vi "CSM.vi"(7 "Name(\"\" to use uuid)":string="csm") -> ()   [LabVIEW 2020]
uses:
  d2b1b62f-1b90-408b-bb7a-e556077d75a7.vi
  8b8ec819-a2be-48ca-834e-c0b9cb0b2cd9.vi
  <userlib>/_NEVSTOP/Communicable State Machine(CSM)/_Support/Common/Format Timestamp.vi
  <userlib>/_NEVSTOP/Communicable State Machine(CSM)/AdvanceAPI/CSM - Revert Arguments-Safe String.vi
  <userlib>/_NEVSTOP/Communicable State Machine(CSM)/_Support/Common/Trim Single line Text.vi
  <userlib>/_NEVSTOP/Communicable State Machine(CSM)/AdvanceAPI/CSM - Make String Arguments Safe.vi
  <userlib>/_NEVSTOP/Communicable State Machine(CSM)/AdvanceAPI/CSM - Break Down Multiple States String.vi
  <userlib>/_NEVSTOP/Communicable State Machine(CSM)/AdvanceAPI/CSM - Compact Multiple States.vi
  <userlib>/_NEVSTOP/Communicable State Machine(CSM)/AdvanceAPI/CSM - Keywords.vi
  <userlib>/_NEVSTOP/Communicable State Machine(CSM)/addons/API-String-Arugments-Support/_Support/Data To API String Arguments.vi
  Global.vi
  <userlib>/_NEVSTOP/Communicable State Machine(CSM)/Communicable State Machine.lvlib
panel:
  out "State History":string
  in  "Init State(\"Macro: Initialize\")":string="Macro: Initialize"
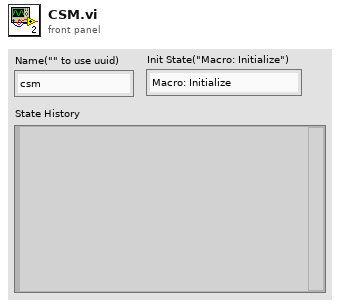
[diagram p1: front panel]
types:
  T1 = enum32{"Invalid", "Standard", "Closed", "Hidden", "Minimized", "Maximized"}
  T2 = enum32{"invalid app kind", "Development System", "Run Time System", "Student Edition", "Embedded LabVIEW", "Evaluation", "Custom"}
  T3 = typedef "Communicable State Machine.lvlib/_CSM_Response Source Message.ctl" = cluster{"‘State":string, "’Arguments":string, "’Error":errorcluster}
  T4 = cluster{"Current VI Reference":refnum<vi>, "Close Panel on Exit?":bool}
  T5 = cluster{"Core":cluster{"Current VI Reference":refnum<vi>, "Close Panel on Exit?":bool}, "num":i32}
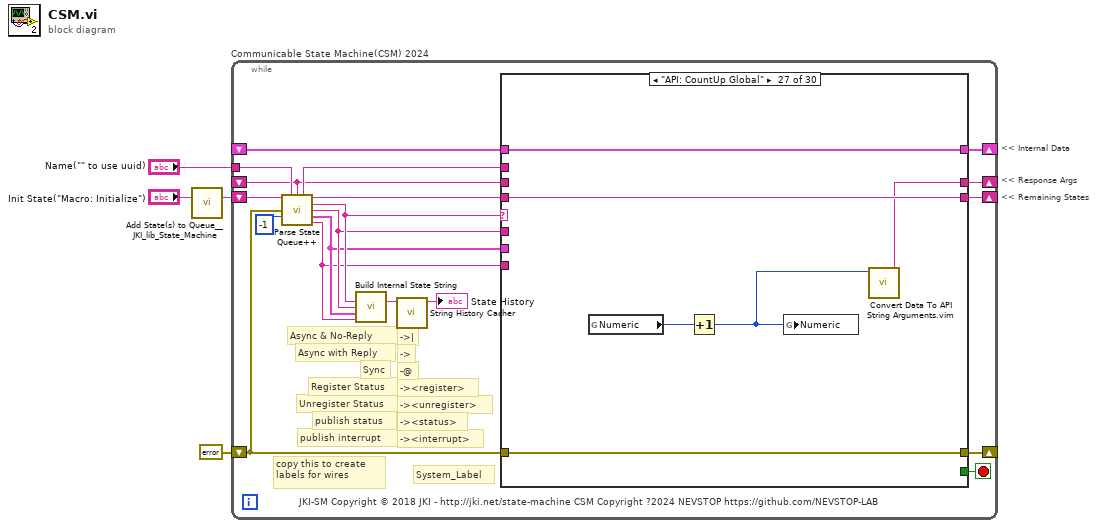
[diagram p0: block diagram]
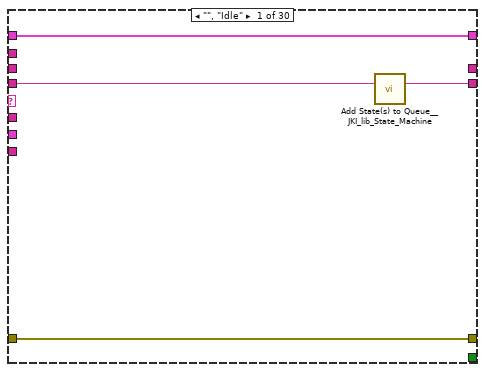
[diagram p2: hidden frame]
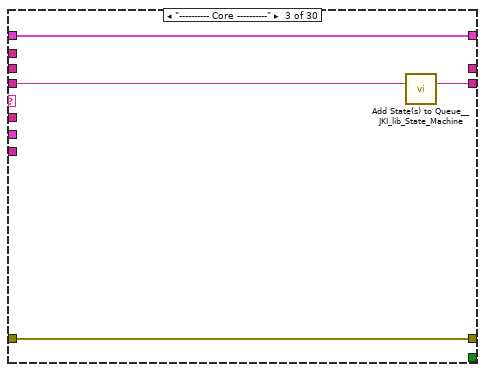
[diagram p4: hidden frame]
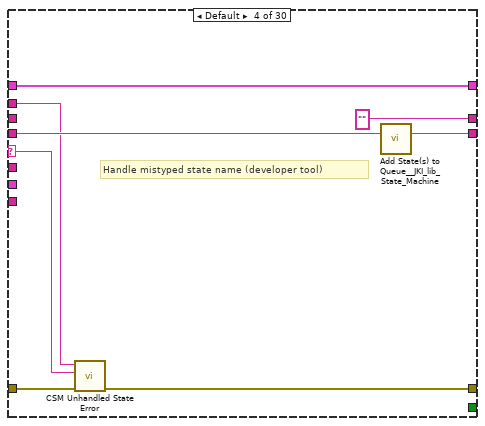
[diagram p5: hidden frame]
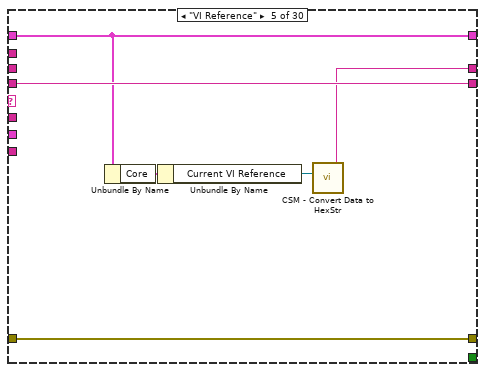
[diagram p6: hidden frame]
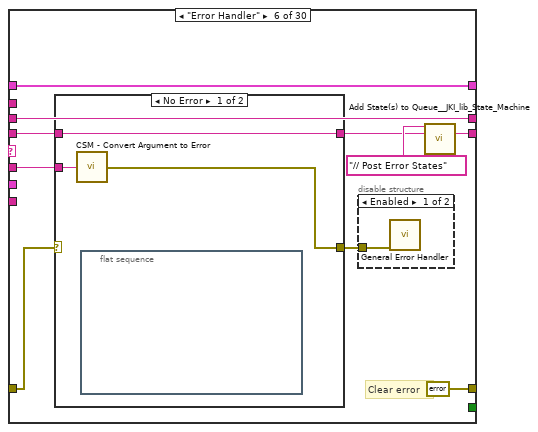
[diagram p7: hidden frame]
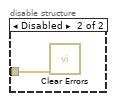
[diagram p8: hidden frame]
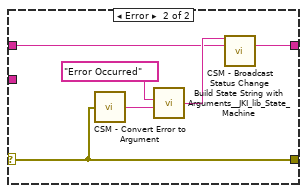
[diagram p9: hidden frame]
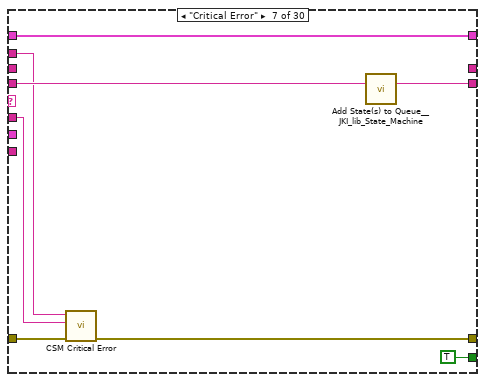
[diagram p10: hidden frame]
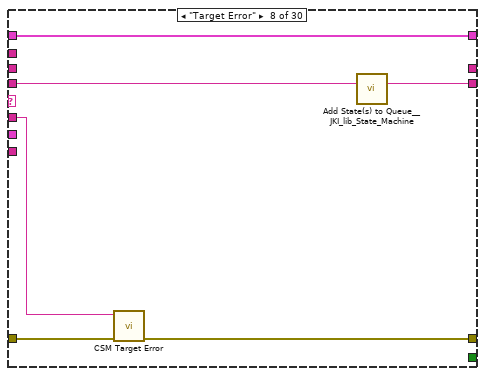
[diagram p11: hidden frame]
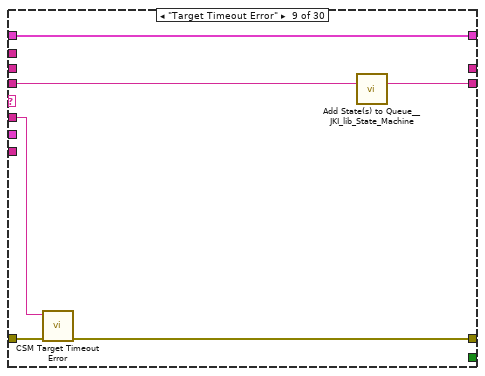
[diagram p12: hidden frame]
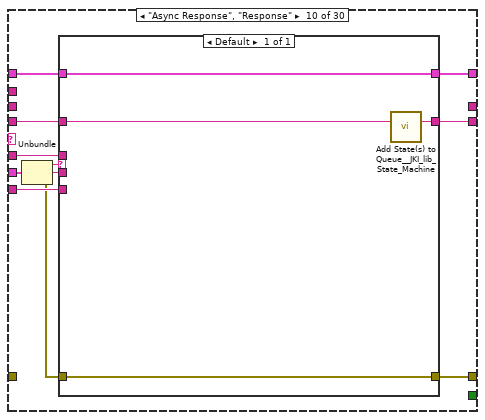
[diagram p13: hidden frame]
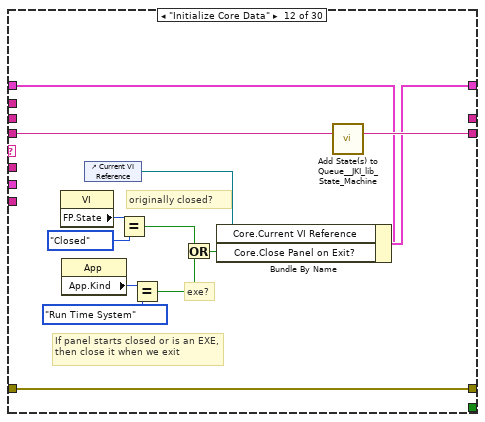
[diagram p15: hidden frame]
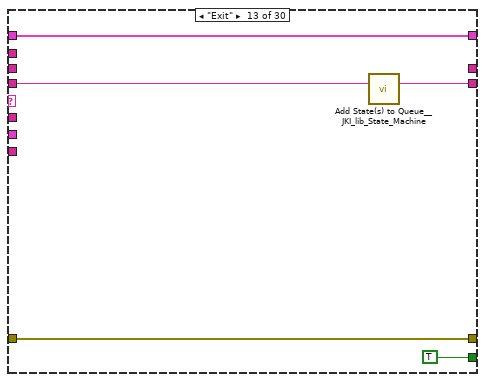
[diagram p16: hidden frame]
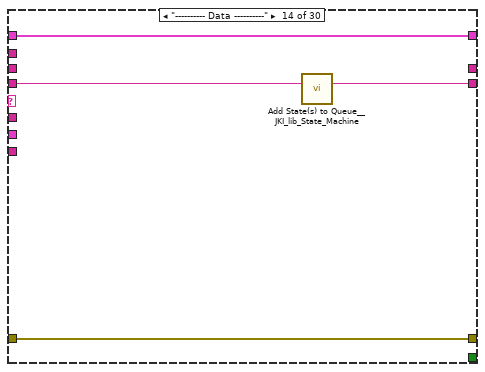
[diagram p17: hidden frame]
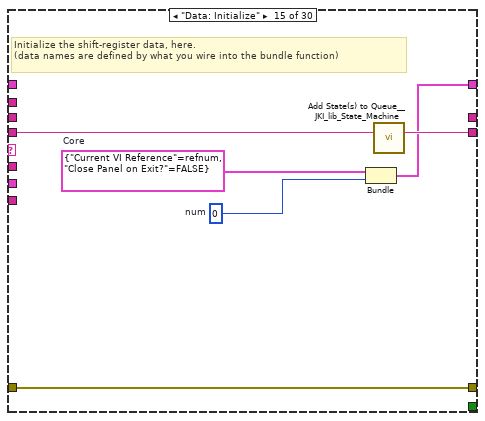
[diagram p18: hidden frame]
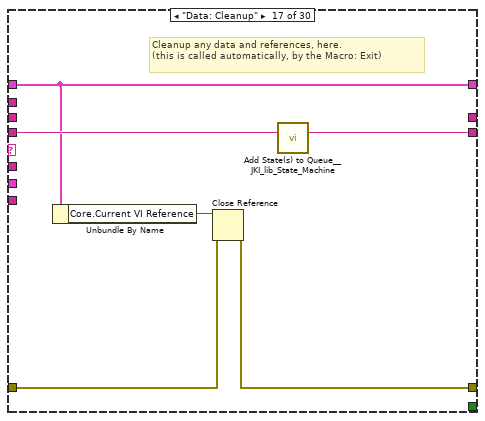
[diagram p20: hidden frame]
diagram:
  # "<< Internal Data"
  # "<< Response Args"
  # "<< Remaining States"
  n1 = call <vilib>:"Add State(s) to Queue__JKI_lib_State_Machine.vi"("State(s) in (\"\")"="Init State(\"Macro: Initialize\")") -> ("States Out"=w1:string)  [unwired: 14 in]
  n2 = while "Communicable State Machine(CSM) 2024" {
    shift-right: [w18] -> _
    shift-left: _ -> [w17]
    shift-right: [w21] -> _
    shift-left: errorcluster {"status"=FALSE, "code"=0, "source"=""} ("error out") -> [w16]
    shift-right: [w20] -> _
    shift-left: w1 -> [w22]
    tunnel: "Name(\"\" to use uuid)" -> [w14]
    shift-right: [w15] -> _
    shift-left: _ -> [w6]
    stop <- w19 stop-if-true
    # "-><interrupt>"
    # "-><status>"
    # "-><unregister>"
    # "-><register>"
    # "-@"
    # "->"
    # "->|"
    # "publish interrupt"
    # "publish status"
    # "Unregister Status"
    # "Register Status"
    # "Sync"
    # "Async with Reply"
    # "Async & No-Reply"
    # "copy this to create labels for wires"
    # "System_Label"
    # "JKI-SM Copyright © 2018 JKI - http://jki.net/state-machine CSM Copyright ?2024 NEVSTOP https://github.com/NEVSTOP-LAB"
    n3 = call <userlib>:"Parse State Queue++.vi"("State Queue"=w22, "Name(\"\" to use uuid)"=w14, "Response Arguments"=w6, "Previous Error"=w16, "Dequeue Timeout(0ms)"=-1 ("Timeout")) -> ("Name Used"=w7:string, "Remaining States"=w23:string, "Current State"=w11:string, "Arguments"=w10:string, ">> Response Source Message >>"=w9:T3, ">> Source CSM >>"=w8:string)  [unwired: 5 in]
    n4 = call <userlib>:"Build Internal State String.vi"("State"=w11, "Arguments (\"\")"=w10, ">> Response Source Message >>"=w9, "Source (\"\")"=w8) -> ("State with Arguments"=w12:string)  [unwired: 11 in]
    n5 = call <userlib>:"String History Cacher.vi"("String"=w12) -> ("String Cache"=→"State History":string)  [unwired: 10 in]
    n6 = case shown="\"API: CountUp Global\"" w11 {
      selector: w11 -> [_ _ _ w37 _ _ _ _ _ _ _ _ _ _ _ _ _ _ _ _ _ _ _ _ _ _ _ _ _ _]
      tunnel: w23 -> [w24 w29 w34 w41 w47 w54 w75 w81 w87 w95 w106 w120 w125 w129 w135 w137 w144 w148 w152 w158 w173 w242 w247 w254 w256 w263 w269 w274 w278 w282]
      tunnel: w10 -> [_ _ _ _ _ w53 w71 w80 w85 w94 _ _ _ _ _ _ _ _ _ w153 w167 _ _ _ _ _ _ _ _ _]
      tunnel: w17 -> [w25 w28 w31 w39 w46 w57 w76 w82 w88 w97 w105 w113 w123 w126 _ w136 w139 w145 w150 w156 w169 w239 w244 w251 w255 w262 w268 w271 w275 w279]
      tunnel: [w26 w30 w32 w35 w48 errorcluster {"status"=FALSE, "code"=0, "source"=""} ("error out") w72 w78 w84 w100 w107 w117 w122 w127 w132 w138 w140 w146 w149 w154 w170 w240 w245 w252 w257 w264 w270 w272 w276 w280] -> w21
      tunnel: w16 -> [w26 w30 w32 w42 w48 w55 w77 w79 w86 _ w107 w117 w122 w127 w132 w138 w141 w146 w149 w155 w171 w240 w245 w252 w257 w264 w270 w272 w276 w280]
      tunnel: [w27 w29 w33 w40 w47 w50 w74 w83 w89 w96 w106 w119 w124 w128 w134 w137 w143 w147 w151 w157 w172 w241 w246 w253 w256 w263 w269 w273 w277 w281] -> w20
      tunnel: [_ _ _ _ _ _ TRUE _ _ _ _ _ TRUE _ _ _ _ _ _ _ _ _ _ _ _ _ _ _ _ _] -> w19
      tunnel: [w25 w28 w31 w39 w46 w57 w76 w82 w88 w98 w105 w118 w123 w126 w133 w136 w139 w145 w150 w156 w169 w239 w244 w251 w255 w260 w268 w271 w275 w279] -> w18
      tunnel: w8 -> [_ _ _ _ _ _ _ _ _ w92 _ _ _ _ _ _ _ _ _ _ _ _ _ _ _ _ _ _ _ _]
      tunnel: w9 -> [_ _ _ _ _ _ _ _ _ w99 _ _ _ _ _ _ _ _ _ _ _ _ _ _ _ _ _ _ _ _]
      tunnel: [_ _ _ "" w43 w49 _ _ _ _ _ _ _ _ _ _ _ _ _ _ _ _ _ _ _ w258 w267 _ _ _] -> w15
      tunnel: w7 -> [_ _ _ w36 _ _ w70 _ _ _ _ _ _ _ _ _ _ _ _ _ _ _ _ _ _ _ _ _ _ _]
      tunnel: w6 -> [_ _ _ _ _ w49 _ _ _ _ _ _ _ _ _ _ _ _ _ _ _ _ _ _ _ _ _ _ _ _]
      frame "", "Idle" {
        n7 = call <vilib>:"Add State(s) to Queue__JKI_lib_State_Machine.vi"("State(s) in (\"\")"=w24) -> ("States Out"=w27:string)  [unwired: 14 in]
      }
      frame "CSM Documentation" {
      }
      frame "---------- Core ----------" {
        n8 = call <vilib>:"Add State(s) to Queue__JKI_lib_State_Machine.vi"("State(s) in (\"\")"=w34) -> ("States Out"=w33:string)  [unwired: 14 in]
      }
      frame Default {
        # "Handle mistyped state name (developer tool)"
        n9 = call <userlib>:"CSM Unhandled State Error.vi"("error in (no error)"=w42, "Current State"=w37, "CSM Name"=w36) -> ("error out"=w35:errorcluster)  [unwired: 8 in]
        n10 = call <vilib>:"Add State(s) to Queue__JKI_lib_State_Machine.vi"("State(s) in (\"\")"=w41) -> ("States Out"=w40:string)  [unwired: 14 in]
      }
      frame "VI Reference" {
        n11 = Unbundle By Name(w46) -> ("Core"=w45:T4)
        n12 = Unbundle By Name(w45) -> ("Current VI Reference"=w44:refnum<vi>)
        n13 = call <userlib>:"CSM - Convert Data to HexStr.vi"("Variant"=w44) -> ("HEX String (0-9,A-F)"=w43:string)  [unwired: 8 in]
      }
      frame "Error Handler" {
        # "Clear error"
        n14 = case shown="No Error" w55 {
          selector: w55 -> [_ w64]
          tunnel: [w63 w66] -> w51
          tunnel: w54 -> [w63 w65]
          tunnel: w53 -> [w62 _]
          tunnel: [w61 w64] -> w56
          frame No Error {
            n15 = call <userlib>:"CSM - Convert Argument to Error.vi"("Argument"=w62) -> ("error"=w61:errorcluster)  [unwired: 4 in]
            n16 = flat-sequence {
              frame #0 {
              }
            }
          }
          frame Error {
            n17 = call <userlib>:"CSM - Convert Error to Argument.vi"("error"=w64) -> ("Argument"=w68:string)  [unwired: 4 in]
            n18 = call <vilib>:"Build State String with Arguments__JKI_lib_State_Machine.vi"("Arguments (\"\")"=w68, "State"="Error Occurred" ("Status with Arguments")) -> ("State with Arguments"=w67:string)  [unwired: 4 in]
            n19 = call <userlib>:"CSM - Broadcast Status Change.vi"("Status with Arguments"=w67, "State Queue"=w65) -> ("Remaining States"=w66:string)  [unwired: 13 in]
          }
        }
        n20 = disable-structure shown="Enabled" {
          disable-tunnel: w56 -> [w59 w60]
          frame Enabled {
            n21 = call <vilib>:"General Error Handler.vi"("error in (no error)"=w59) -> ()  [unwired: 10 in, 5 out]
          }
          frame Disabled {
            n22 = call <vilib>:"Clear Errors.vi"("error in (no error)"=w60) -> ()  [unwired: 5 in, 2 out]
          }
        }
        n23 = call <vilib>:"Add State(s) to Queue__JKI_lib_State_Machine.vi"("State(s) in Front (\"\")"="// Post Error States", "State(s) in (\"\")"=w51) -> ("States Out"=w50:string)  [unwired: 13 in]
      }
      frame "Critical Error" {
        n24 = call <userlib>:"CSM Critical Error.vi"("error in (no error)"=w77, "Arugments(as Reason)"=w71, "CSM Name"=w70) -> ("error out"=w72:errorcluster)  [unwired: 8 in]
        n25 = call <vilib>:"Add State(s) to Queue__JKI_lib_State_Machine.vi"("State(s) in (\"\")"=w75) -> ("States Out"=w74:string)  [unwired: 14 in]
      }
      frame "Target Error" {
        n26 = call <userlib>:"CSM Target Error.vi"("error in (no error)"=w79, "Arguments(as CSM Name)"=w80) -> ("error out"=w78:errorcluster)  [unwired: 9 in]
        n27 = call <vilib>:"Add State(s) to Queue__JKI_lib_State_Machine.vi"("State(s) in (\"\")"=w81) -> ("States Out"=w83:string)  [unwired: 14 in]
      }
      frame "Target Timeout Error" {
        n28 = call <userlib>:"CSM Target Timeout Error.vi"("error in (no error)"=w86, "Arguments(as CSM Name)"=w85) -> ("error out"=w84:errorcluster)  [unwired: 9 in]
        n29 = call <vilib>:"Add State(s) to Queue__JKI_lib_State_Machine.vi"("State(s) in (\"\")"=w87) -> ("States Out"=w89:string)  [unwired: 14 in]
      }
      frame "Async Response", "Response" {
        n30 = Unbundle(w99) -> ("‘State"=w93:string, "’Arguments"=w91:string, "’Error"=w90:errorcluster)
        n31 = case shown="Default" w93 {
          tunnel: [w104] -> w100
          tunnel: w90 -> [w104]
          tunnel: [w103] -> w98
          tunnel: w97 -> [w103]
          tunnel: [w101] -> w96
          tunnel: w95 -> [w102]
          tunnel: w94 -> [_]
          tunnel: w92 -> [_]
          tunnel: w91 -> [_]
          frame Default {
            n32 = call <vilib>:"Add State(s) to Queue__JKI_lib_State_Machine.vi"("State(s) in (\"\")"=w102) -> ("States Out"=w101:string)  [unwired: 14 in]
          }
        }
      }
      frame "Async Message Posted" {
      }
      frame "Initialize Core Data" {
        # "originally closed?"
        # "exe?"
        # "If panel starts closed or is an EXE, then close it when we exit"
        n33 = property class="VI"() -> ("FP.State"=w110:T1)  [unwired: 2 in, 2 out]
        n34 = property class="App"() -> ("App.Kind"=w116:T2)  [unwired: 2 in, 2 out]
        n35 = control-ref of="Current VI Reference"() -> (w111:refnum<vi>)
        n36 = Equal?(x=w110, y=T1."Closed" ("Front Panel Window:State")) -> (x = y?=w108:bool)
        n37 = Equal?(x=w116, y=T2."Run Time System" ("Application:Kind")) -> (x = y?=w114:bool)
        n38 = Or(x=w108, y=w114) -> (x .or. y?=w112:bool)
        n39 = Bundle By Name(cluster=w113, "Core.Current VI Reference"=w111, "Core.Close Panel on Exit?"=w112) -> (w118:T5)
        n40 = call <vilib>:"Add State(s) to Queue__JKI_lib_State_Machine.vi"("State(s) in (\"\")"=w120) -> ("States Out"=w119:string)  [unwired: 14 in]
      }
      frame "Exit" {
        n41 = call <vilib>:"Add State(s) to Queue__JKI_lib_State_Machine.vi"("State(s) in (\"\")"=w125) -> ("States Out"=w124:string)  [unwired: 14 in]
      }
      frame "---------- Data ----------" {
        n42 = call <vilib>:"Add State(s) to Queue__JKI_lib_State_Machine.vi"("State(s) in (\"\")"=w129) -> ("States Out"=w128:string)  [unwired: 14 in]
      }
      frame "Data: Initialize" {
        w130 = T4 {"Current VI Reference"=refnum, "Close Panel on Exit?"=FALSE}  # Core
        w131 = 0  # num
        # "Initialize the shift-register data, here.\n(data names are defined by what you wire into the bundle function)"
        n43 = Bundle("Core"=w130, "num"=w131) -> (w133:T5)  [unwired: 1 in]
        n44 = call <vilib>:"Add State(s) to Queue__JKI_lib_State_Machine.vi"("State(s) in (\"\")"=w135) -> ("States Out"=w134:string)  [unwired: 14 in]
      }
      frame "Data: Update Indicators" {
      }
      frame "Data: Cleanup" {
        # "Cleanup any data and references, here.\n(this is called automatically, by the Macro: Exit)"
        n45 = Unbundle By Name(w139) -> ("Core.Current VI Reference"=w142:refnum<vi>)
        n46 = Close Reference(reference=w142, error in (no error)=w141) -> (error out=w140:errorcluster)
        n47 = call <vilib>:"Add State(s) to Queue__JKI_lib_State_Machine.vi"("State(s) in (\"\")"=w144) -> ("States Out"=w143:string)  [unwired: 14 in]
      }
      frame "---------- UI ----------" {
        n48 = call <vilib>:"Add State(s) to Queue__JKI_lib_State_Machine.vi"("State(s) in (\"\")"=w148) -> ("States Out"=w147:string)  [unwired: 14 in]
      }
      frame "UI: Initialize" {
        n49 = call <vilib>:"Add State(s) to Queue__JKI_lib_State_Machine.vi"("State(s) in (\"\")"=w152) -> ("States Out"=w151:string)  [unwired: 14 in]
      }
      frame "UI: Cursor Set" {
        # "Argument"
        n50 = disable-structure shown="TARGET_TYPE!=Windows" {
          disable-tunnel: w155 -> [w161 w166]
          disable-tunnel: [w160 w166] -> w154
          disable-tunnel: w153 -> [w159 _]
          frame condition #0 (active) {
            n51 = case shown="\"Idle\", Default" w159 {
              tunnel: w161 -> [w163 w165]
              tunnel: [w162 w164] -> w160
              frame "Idle", Default {
                n52 = call <vilib>:"Unset Busy.vi"("error in (no error)"=w163) -> ("error out"=w162:errorcluster)  [unwired: 10 in]
              }
              frame "Busy" {
                n53 = call <vilib>:"Set Busy.vi"("error in (no error)"=w165) -> ("error out"=w164:errorcluster)  [unwired: 9 in, 1 out]
              }
            }
          }
          frame condition #1 {
          }
        }
        n54 = call <vilib>:"Add State(s) to Queue__JKI_lib_State_Machine.vi"("State(s) in (\"\")"=w158) -> ("States Out"=w157:string)  [unwired: 14 in]
      }
      frame "UI: Front Panel State" {
        # "Argument"
        n55 = Unbundle By Name(w169) -> ("Core.Current VI Reference"=w168:refnum<vi>)
        n56 = call <vilib>:"Add State(s) to Queue__JKI_lib_State_Machine.vi"("State(s) in (\"\")"=w173) -> ("States Out"=w172:string)  [unwired: 14 in]
        n57 = case shown="\"Close\", \"Closed\"" w167 {
          tunnel: w171 -> [w179 w194 w205 w218 w231]
          tunnel: [w181 w195 w207 w220 w233] -> w170
          tunnel: w168 -> [w180 w192 w206 w219 w232]
          frame "Open", "Standard", Default {
            w174 = T1."Standard" ("State")
            n58 = property class="VI"(reference=w180, error in=w179) -> (reference out=w177:refnum<vi>, error out=w178:errorcluster, "FP.State"=w176:T1)
            n59 = Not Equal?(x=w176, y=w174) -> (x != y?=w175:bool)
            n60 = case shown="True" w175 {
              tunnel: [w185 w187] -> w181
              tunnel: w178 -> [w184 w187]
              tunnel: w177 -> [w183 _]
              tunnel: w174 -> [w182 _]
              frame True {
                n61 = invoke class="VI" method="FP.Open"(reference=w183, error in=w184, "Activate"=TRUE, "State"=w182) -> (error out=w185:errorcluster)  [unwired: 1 in, 4 out]
              }
              frame False {
              }
            }
          }
          frame "Close", "Closed" {
            n62 = property class="VI"(reference=w192, error in=w194) -> (reference out=w191:refnum<vi>, error out=w193:errorcluster, "FP.State"=w189:T1)
            n63 = Not Equal?(x=w189, y=T1."Closed" ("Front Panel Window:State")) -> (x != y?=w188:bool)
            n64 = case shown="False" w188 {
              tunnel: [w196 w199] -> w195
              tunnel: w193 -> [w196 w198]
              tunnel: w191 -> [_ w197]
              frame False {
              }
              frame True {
                n65 = invoke class="VI" method="FP.Close"(reference=w197, error in=w198) -> (error out=w199:errorcluster)  [unwired: 1 in, 2 out]
              }
            }
          }
          frame "Hidden", "Hide" {
            w200 = T1."Hidden" ("State")
            n66 = property class="VI"(reference=w206, error in=w205) -> (reference out=w203:refnum<vi>, error out=w204:errorcluster, "FP.State"=w202:T1)
            n67 = Not Equal?(x=w202, y=w200) -> (x != y?=w201:bool)
            n68 = case shown="True" w201 {
              tunnel: [w211 w212] -> w207
              tunnel: w204 -> [w210 w212]
              tunnel: w203 -> [w209 _]
              tunnel: w200 -> [w208 _]
              frame True {
                n69 = invoke class="VI" method="FP.Open"(reference=w209, error in=w210, "State"=w208) -> (error out=w211:errorcluster)  [unwired: 2 in, 4 out]
              }
              frame False {
              }
            }
          }
          frame "Minimize", "Minimized" {
            w213 = T1."Minimized" ("State")
            n70 = property class="VI"(reference=w219, error in=w218) -> (reference out=w216:refnum<vi>, error out=w217:errorcluster, "FP.State"=w215:T1)
            n71 = Not Equal?(x=w215, y=w213) -> (x != y?=w214:bool)
            n72 = case shown="True" w214 {
              tunnel: [w224 w225] -> w220
              tunnel: w217 -> [w223 w225]
              tunnel: w216 -> [w222 _]
              tunnel: w213 -> [w221 _]
              frame True {
                n73 = invoke class="VI" method="FP.Open"(reference=w222, error in=w223, "State"=w221) -> (error out=w224:errorcluster)  [unwired: 2 in, 4 out]
              }
              frame False {
              }
            }
          }
          frame "Maximize", "Maximized" {
            w226 = T1."Maximized" ("State")
            n74 = property class="VI"(reference=w232, error in=w231) -> (reference out=w229:refnum<vi>, error out=w230:errorcluster, "FP.State"=w228:T1)
            n75 = Not Equal?(x=w228, y=w226) -> (x != y?=w227:bool)
            n76 = case shown="True" w227 {
              tunnel: [w237 w238] -> w233
              tunnel: w230 -> [w236 w238]
              tunnel: w229 -> [w235 _]
              tunnel: w226 -> [w234 _]
              frame True {
                n77 = invoke class="VI" method="FP.Open"(reference=w235, error in=w236, "State"=w234) -> (error out=w237:errorcluster)  [unwired: 2 in, 4 out]
              }
              frame False {
              }
            }
          }
        }
      }
      frame "---------- Macro ----------" {
        n78 = call <vilib>:"Add State(s) to Queue__JKI_lib_State_Machine.vi"("State(s) in (\"\")"=w242) -> ("States Out"=w241:string)  [unwired: 14 in]
      }
      frame "Macro: Initialize" {
        n79 = call <vilib>:"Add State(s) to Queue__JKI_lib_State_Machine.vi"("State(s) in Front (\"\")"="Data: Initialize\nInitialize Core Data\nData: Update Indicators", "State(s) in (\"\")"=w247) -> ("States Out"=w246:string)  [unwired: 13 in]
      }
      frame "Macro: Exit" {
        n80 = call <vilib>:"Add State(s) to Queue__JKI_lib_State_Machine.vi"("State(s) in Front (\"\")"="//Exit Sub-Modules ", "State(s) at Back (\"\")"="Data: Cleanup\nExit") -> ("States Out"=w249:string)  [unwired: 13 in]
        n81 = call <vilib>:"Add State(s) to Queue__JKI_lib_State_Machine.vi"("State(s) in Front (\"\")"=w249, "State(s) in (\"\")"=w254) -> ("States Out"=w253:string)  [unwired: 13 in]
      }
      frame "---------- API ----------" {
      }
      frame "API: CountUp" {
        n82 = Unbundle By Name(w262) -> ("num"=w261:i32)
        n83 = Increment(x=w261) -> (x+1=w259:i32)
        n84 = Bundle By Name(cluster=w262, "num"=w259) -> (w260:T5)
        n85 = call "Convert Data To API String Arguments.vim"("data"=w259) -> ("String"=w258:string)  [unwired: 7 in, 1 out]
      }
      frame "API: CountUp Global" {
        n86 = global read "Global.vi" "Numeric"() -> (w266:i32)
        n87 = Increment(x=w266) -> (x+1=w265:i32)
        n88 = global write "Global.vi" "Numeric"(w265) -> ()
        n89 = call "Convert Data To API String Arguments.vim"("data"=w265) -> ("String"=w267:string)  [unwired: 7 in, 1 out]
      }
      frame "---------- Action ----------" {
        n90 = call <vilib>:"Add State(s) to Queue__JKI_lib_State_Machine.vi"("State(s) in (\"\")"=w274) -> ("States Out"=w273:string)  [unwired: 14 in]
      }
      frame "Action: action1" {
        n91 = call <vilib>:"Add State(s) to Queue__JKI_lib_State_Machine.vi"("State(s) in (\"\")"=w278) -> ("States Out"=w277:string)  [unwired: 14 in]
      }
      frame "Action: action2" {
        n92 = call <vilib>:"Add State(s) to Queue__JKI_lib_State_Machine.vi"("State(s) in (\"\")"=w282) -> ("States Out"=w281:string)  [unwired: 14 in]
      }
    }
  }
